vi "Launch Subordinate.vi"(8 "error in":errorcluster, 9 "Panel Definiton":T2, 10 "Identifier":string, 11 "Manual UI in":refnum<class "Manual UI.lvclass">) -> (0 "error out":errorcluster, 2 "Subordinate":T1, 3 "Manual UI out":refnum<class "Manual UI.lvclass">)   [LabVIEW 2023, in "Manual UI.lvlib" / "Manual UI.lvclass"]
uses:
  Project/Manual UI.lvclass
  builds/Engine/Panel Manager.lvlibp/Panel Actor/Panel Actor.lvclass
  C:/Users/Public/Documents/Development/builds/Engine/Actor Framework.lvlibp/1abvi3w/vi.lib/ActorFramework/Actor/Actor.lvclass
  builds/Engine/Panel.lvlibp/Panel/Panel.lvclass
  builds/Engine/Actor Framework.lvlibp/1abvi3w/vi.lib/ActorFramework/Message Enqueuer/Message Enqueuer.lvclass
  builds/Engine/Actor Framework.lvlibp/1abvi3w/vi.lib/ActorFramework/Actor/Write Actor Label.vi
  C:/Users/Public/Documents/Development/builds/Engine/Panel Manager.lvlibp/Panel Actor/Panel Actor.lvclass
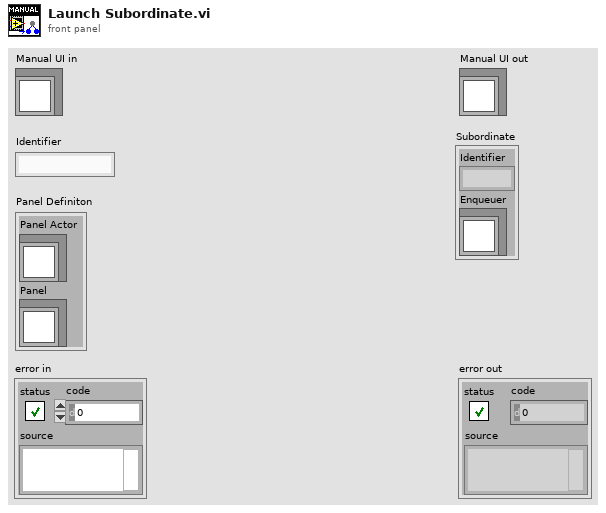
[diagram p1: front panel]
types:
  T1 = cluster{"Identifier":string, "Enqueuer":refnum<class "Message Enqueuer.lvclass">}
  T2 = cluster{"Panel Actor":refnum<class "Panel Actor.lvclass">, "Panel":refnum<class "Panel.lvclass">}
  T3 = cluster{"Identifier":string, "Nested Actor's Enqueuer":refnum<class "Message Enqueuer.lvclass">}
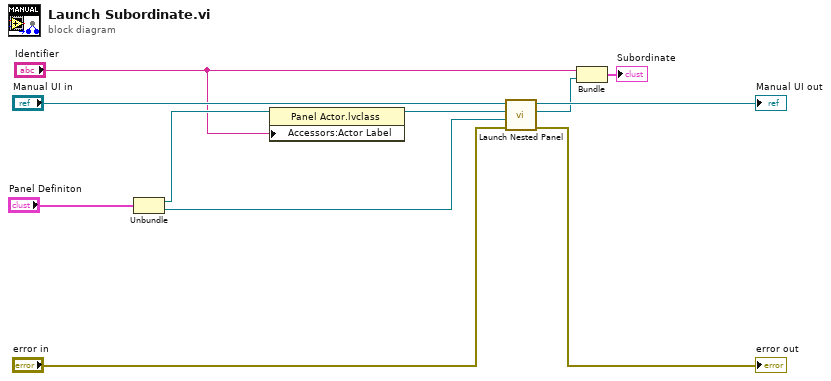
[diagram p0: block diagram]
diagram:
  n1 = Unbundle("Panel Definiton") -> ("Panel Actor"=w10:refnum<class "Panel Actor.lvclass">, "Panel"=w6:refnum<class "Panel.lvclass">)
  n2 = property class="Panel Actor.lvclass"(reference=w10, "Accessors:Actor Label"="Identifier") -> (reference out=w7:refnum<class "Panel Actor.lvclass">)  [unwired: 1 in, 1 out]
  n3 = call "Launch Nested Panel.vi"("error in (no error)"="error in", "Panel"=w6, "Nested Panel Actor"=w7, "Panel Actor in"="Manual UI in") -> ("error out"=→"error out":errorcluster, "Nested Actor's Enqueuer"=w3:refnum<class "Message Enqueuer.lvclass">, "Panel Actor out"=→"Manual UI out":refnum<class "Manual UI.lvclass">)  [unwired: 4 in, 1 out]
  n4 = Bundle("Identifier"="Identifier", "Nested Actor's Enqueuer"=w3) -> (→"Subordinate":T3)  [unwired: 1 in]
